vi "Begin.vi"(8 "error in":errorcluster) -> (0 "error out":errorcluster)   [LabVIEW 2015]
doc: "Called before other user functions, this VI is expected to open initial I/O refnums, load in file data, and do all program initialization. Notice that the <B>error out</B> terminal is simply used for data flow. Wiring it to other structures or subVIs ensures that this VI runs first."
uses:
  <vilib>/Rock Robotics/SystemInterfaces/i2clib/i2c_bus.ctl
  <vilib>/Rock Robotics/WPI/I2C/WPI_I2CDevRef.ctl
  <vilib>/Rock Robotics/WPI/DriverStation/WPI_DriverStationRobotMode2.ctl
  <vilib>/Rock Robotics/WPI/Joystick/WPI_JoystickDeviceEnum.ctl
  <vilib>/Rock Robotics/SystemInterfaces/AI/FPGA_AIGyroChannel.ctl
  <vilib>/Rock Robotics/WPI/Accelerometer/WPI_AccelerometerRange.ctl
  <vilib>/Rock Robotics/WPI/Solenoid/WPI_SolenoidChannel.ctl
  <vilib>/Rock Robotics/SystemInterfaces/DIO/FPGA_DIOChannel.ctl
  <vilib>/Rock Robotics/SystemInterfaces/DIO/FPGA_DIOPWMChannel.ctl
  <vilib>/Rock Robotics/SystemInterfaces/AI/FPGA_AIChannel.ctl
  <vilib>/Rock Robotics/WPI/CAN/TalonSRX/WPI_CANTalonSRX_BrakeOverride.ctl
  Robot Global Data.vi
  <vilib>/Rock Robotics/WPI/Gyro/WPI_GyroAnalogOpen.vi
  <vilib>/Rock Robotics/WPI/Accelerometer/InternalAccelerometer/WPI_AccelerometerInternalOpen.vi
  <vilib>/Rock Robotics/WPI/Solenoid/WPI_SolenoidOpenDouble.vi
  <vilib>/Rock Robotics/WPI/Counter/WPI_CounterDigitalInputToDigitalSource.vi
  <vilib>/Rock Robotics/WPI/MotorControl/WPI_MotorControlOpen Talon.vi
  <vilib>/Rock Robotics/WPI/MotorControl/WPI_MotorControlOpenCANTalonSRX.vi
  <vilib>/Rock Robotics/WPI/RobotDrive/WPI_RobotDriveOpen4MotorWithCANTalonSRX.vi
  <vilib>/Rock Robotics/WPI/RobotDrive/WPI_RobotDriveOpen2MotorWithTalon.vi
panel:
  in  "Alt Adr":bool=TRUE
  in  "Flash Drive? 2":bool
  out "I2CDevRef out 2":T1={"DevStatus"={"status"=FALSE, "code"=0, "source"=""}, "Device Address"=40, "Handle"=45, "I2C Bus"=enum."I2C MXP"} {"Device Address" format="%.0x"}
  out "Fatal Result 2":bool
  out "Bad result 2":bool
  in  "Calibrate? 2":bool
  in  "Status delay 2":i32=30
  in  "I2C Bus 2":T2=enum."I2C MXP"
  in  "Placement 2":T3(ring)=enum."P3"
  in  "Op Mode 2":T4(ring)=enum."IMU"
  out "M 2":T5={"Boolean"=TRUE, "Boolean 2"=FALSE, "Boolean 3"=FALSE, "Boolean 4"=FALSE}
  out "A 2":T5={"Boolean"=TRUE, "Boolean 2"=FALSE, "Boolean 3"=FALSE, "Boolean 4"=FALSE}
  out "G 2":T5={"Boolean"=TRUE, "Boolean 2"=FALSE, "Boolean 3"=FALSE, "Boolean 4"=FALSE}
  out "S 2":T5={"Boolean"=TRUE, "Boolean 2"=FALSE, "Boolean 3"=FALSE, "Boolean 4"=FALSE}
  in  "Flash Drive?":bool
  out "I2CDevRef out":T1={"DevStatus"={"status"=FALSE, "code"=0, "source"=""}, "Device Address"=40, "Handle"=45, "I2C Bus"=enum."I2C MXP"} {"Device Address" format="%.0x"}
  out "Fatal Result":bool
  out "Bad result":bool
  out "M":T5={"Boolean"=TRUE, "Boolean 2"=FALSE, "Boolean 3"=FALSE, "Boolean 4"=FALSE}
  out "A":T5={"Boolean"=TRUE, "Boolean 2"=FALSE, "Boolean 3"=FALSE, "Boolean 4"=FALSE}
  out "G":T5={"Boolean"=TRUE, "Boolean 2"=FALSE, "Boolean 3"=FALSE, "Boolean 4"=FALSE}
  out "S":T5={"Boolean"=TRUE, "Boolean 2"=FALSE, "Boolean 3"=FALSE, "Boolean 4"=FALSE}
  in  "Calibrate?":bool
  in  "Status delay":i32=30
  in  "I2C Bus":T2=enum."I2C MXP"
  in  "Placement":T3(ring)=enum."P3"
  in  "Op Mode":T4(ring)=enum."IMU"
  # "C-BOT:"
  # "BNO055 Cal MC P3 01-29-2016 142659"
  # "Alt IMU CBOT CHAMPS: BNO055 Cal M8 P3 04-27-2016 180927"
  # "P-BOT;"
  # "BNO055 Cal MC P3 02-26-2016 205524"
  # "CBOT CHAMPS Pri: BNO055 Cal M8 P3 04-27-2016 181522"
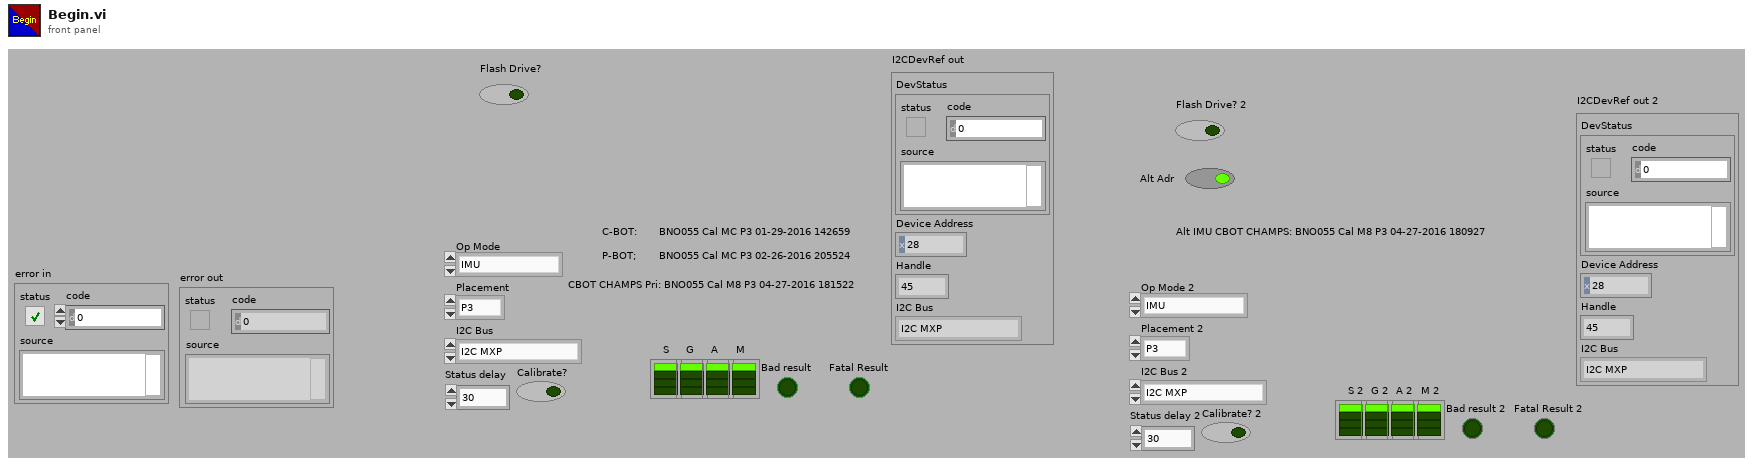
[diagram p1: front panel]
types:
  T1 = typedef "WPI_I2CDevRef.ctl" = cluster{"DevStatus":errorcluster, "Device Address":u8, "Handle":i32, "I2C Bus":T2}
  T2 = typedef "i2c_bus.ctl" = enum16{"I2C On-Board", "I2C MXP", "Invalid"}
  T3 = enum32{"P0", "P1", "P2", "P3", "P4", "P5", "P6", "P7"}
  T4 = enum8{"ConfigMode", "AccOnly", "MagOnly", "GyroOnly", "AccMag", "AccGyro", "MagGyro", "AMG", "IMU", "Compass", "M4G", "NDOF_FMC_OFF", "NDOF"}
  T5 = cluster{"Boolean":bool, "Boolean 2":bool, "Boolean 3":bool, "Boolean 4":bool}
  T6 = typedef "FPGA_DIOPWMChannel.ctl" = enum8{"PWM 0", "PWM 1", "PWM 2", "PWM 3", "PWM 4", "PWM 5", "PWM 6", "PWM 7", "PWM 8", "PWM 9", "PWM MXP 0", "PWM MXP 1", "PWM MXP 2", "PWM MXP 3", "PWM MXP 4", "PWM MXP 5", "PWM MXP 6", "PWM MXP 7", "PWM MXP 8", "PWM MXP 9", "Invalid"}
  T7 = typedef "WPI_SolenoidChannel.ctl" = enum8{"Solenoid 0", "Solenoid 1", "Solenoid 2", "Solenoid 3", "Solenoid 4", "Solenoid 5", "Solenoid 6", "Solenoid 7", "Invalid"}
  T8 = typedef "FPGA_AIChannel.ctl" = enum8{"AI 0", "AI 1", "AI 2", "AI 3", "AI MXP 0", "AI MXP 1", "AI MXP 2", "AI MXP 3", "Invalid"}
  T9 = typedef "FPGA_AIGyroChannel.ctl" = enum8{"AI 0", "AI 1", "Invalid"}
  T10 = typedef "WPI_JoystickDeviceEnum.ctl" = enum16{"USB 0", "USB 1", "USB 2", "USB 3", "USB 4", "USB 5"}
  T11 = typedef "FPGA_DIOChannel.ctl" = enum8{"DIO 0", "DIO 1", "DIO 2", "DIO 3", "DIO 4", "DIO 5", "DIO 6", "DIO 7", "DIO 8", "DIO 9", "DIO MXP 0", "DIO MXP 1", "DIO MXP 2", "DIO MXP 3", "DIO MXP 4", "DIO MXP 5", "DIO MXP 6", "DIO MXP 7", "DIO MXP 8", "DIO MXP 9", "DIO MXP 10", "DIO MXP 11", "DIO MXP 12", "DIO MXP 13", "DIO MXP 14", "DIO MXP 15", "Invalid"}
  T12 = typedef "WPI_AccelerometerRange.ctl" = enum16{"+/- 2 g", "+/- 4 g", "+/- 8 g"}
  T13 = typedef "WPI_DriverStationRobotMode2.ctl" = enum16{"Autonomous Disabled", "Autonomous Enabled", "Teleop Disabled", "Teleop Enabled", "Disconnected", "Finish", "Test Disabled", "Test Enabled", "Emergency Stopped"}
  T14 = typedef "WPI_CANTalonSRX_BrakeOverride.ctl" = enum8{"No Override", "Override to Coast", "Override to Brake"}
  T15 = typedef "WPI_MotorControlDeviceRef.ctl" = cluster{"DeviceStatus":errorcluster, "Type":T16, "PWM":cluster{"PWM Channel":T6, "DeadBand":T17}, "CAN":cluster{"Device Number":u8, "Control Mode":T18, "Semaphore":T19, "Max Vout":dbl, "TalonSRX Control Mode":T20}, "Invert":bool}
  T16 = typedef "WPI_MotorControlType.ctl" = enum16{"PWM", "CAN", "CANTalonSRX"}
  T17 = typedef "WPI_PWMDeadband.ctl" = cluster{"Name":string, "maxPositivePwm":i32, "minPositivePwm":i32, "centerPwm":i32, "maxNegativePwm":i32, "minNegativePwm":i32, "angularRange":u16}
  T18 = typedef "WPI_CANJaguar_ControlMode.ctl" = enum8{"Percent VBus", "Current", "Speed", "Position", "Voltage"}
  T19 = typedef "Semaphore RefNum" = refnum<k1>
  T20 = typedef "WPI_CANTalonSRX_APIControlMode.ctl" = enum8{"Percent VBus", "Speed", "Position", "Slave", "Unchanged / Invalid", "Voltage Compensation", "Current", "Motion Profile"}
  T21 = typedef "WPI_RobotDriveDevRef.ctl" = cluster{"DevStatus":errorcluster, "Motors[]":T15[], "Square Inputs":bool, "Max Output":dbl}
  T22 = typedef "WPI_AccelerometerDevRef.ctl" = cluster{"DevStatus":errorcluster, "Scaling":T23, "Analog Channels":T24, "I2C Bus":T2, "SPI Bus":T25, "Accel Range":T26, "ADXL Axes":T27, "Handle":i32, "Device Address":u8, "Accel Type":enum16{"Analog", "ADXL345 I2C", "ADXL345 SPI", "Internal", "ADXL362 SPI"}}
  T23 = typedef "WPI_AccelerometerScaling.ctl" = cluster{"Gain (VoltsPerG)":dbl, "Center Voltage":dbl}
  T24 = typedef "WPI_AccelerometerAnalogChannels.ctl" = cluster{"X-Axis":T8, "Y-Axis":T8, "Z-Axis":T8}
  T25 = typedef "spi_bus.ctl" = enum16{"SPI On-Board, CS0", "SPI On-Board, CS1", "SPI On-Board, CS2", "SPI On-Board, CS3", "SPI MXP", "Invalid"}
  T26 = typedef "ADXL345 Range.ctl" = u8
  T27 = typedef "WPI_AccelerometerADXL345 Axes.ctl" = cluster{"X-Axis":bool, "Y-Axis":bool, "Z-Axis":bool}
  T28 = typedef "WPI_DigitalInputDevRef.ctl" = cluster{"DevStatus":errorcluster, "DIO Channel":T11}
  T29 = typedef "FPGA_CounterEncoderSourceConvertionLVSourceType.ctl" = cluster{"DevStatus":errorcluster, "AnalogTriggerMode?":bool, "DigitalMode":cluster{"DIO Channel":T30}, "AnalogTriggerMode":cluster{"AnalogTriggerIndex":T31, "OutputType":T32}}
  T30 = typedef "FPGA_DIODigitalSourceChannel.ctl" = enum8{"DIO 0", "DIO 1", "DIO 2", "DIO 3", "DIO 4", "DIO 5", "DIO 6", "DIO 7", "DIO 8", "DIO 9", "DIO MXP 0", "DIO MXP 1", "DIO MXP 2", "DIO MXP 3", "DIO MXP 4", "DIO MXP 5", "DIO MXP 6", "DIO MXP 7", "DIO MXP 8", "DIO MXP 9", "DIO MXP 10", "DIO MXP 11", "DIO MXP 12", "DIO MXP 13", "DIO MXP 14", "DIO MXP 15", "Disabled"}
  T31 = typedef "FPGA_AnalogTriggerIndex.ctl" = enum8{"Trig 0", "Trig 1", "Trig 2", "Trig 3", "Trig 4", "Trig 5", "Trig 6", "Trig 7", "Invalid"}
  T32 = typedef "FPGA_AnalogTriggerOutType.ctl" = enum16{"InWindow", "TriggerState", "Rising", "Falling"}
  T33 = typedef "WPI_EncoderDevRef.ctl" = cluster{"DevStatus":errorcluster, "EncoderIndex":T34, "CounterIndex":T35, "DistancePerCount":dbl, "Decoding Type":T36}
  T34 = typedef "FPGA_EncoderIdx.ctl" = enum8{"Enc 0", "Enc 1", "Enc 2", "Enc 3", "Enc 4", "Enc 5", "Enc 6", "Enc 7", "Invalid"}
  T35 = typedef "FPGA_CounterCtrSystemIndex.ctl" = enum8{"Ctr 0", "Ctr 1", "Ctr 2", "Ctr 3", "Ctr 4", "Ctr 5", "Ctr 6", "Ctr 7", "Invalid"}
  T36 = typedef "WPI_EncoderType.ctl" = enum16{"1x", "2x", "4x"}
  T37 = cluster{"Cluster":cluster{"[0]":bool, "[1]":bool, "[2]":bool, "[3]":bool}, "Cluster":cluster{"[0]":bool, "[1]":bool, "[2]":bool, "[3]":bool}, "Cluster":cluster{"[0]":bool, "[1]":bool, "[2]":bool, "[3]":bool}, "Cluster":cluster{"[0]":bool, "[1]":bool, "[2]":bool, "[3]":bool}}
  T38 = cluster{"[0]":bool, "[1]":bool, "[2]":bool, "[3]":bool}
  T39 = typedef "WPI_JoystickDevRef.ctl" = cluster{"Device":T10}
  T40 = typedef "WPI_SolenoidDevRef.ctl" = cluster{"DevStatus":errorcluster, "Pneumatics Control Module":u8, "Forward Solenoid Channel":T7, "Reverse Solenoid Channel":T7}
  T41 = typedef "WPI_GyroDevRef.ctl" = cluster{"DevStatus":errorcluster, "Analog Channel":T8, "Offset":dbl, "Gain (VoltsPerDegree/Second)":dbl, "Gyro Type":enum16{"Analog", "XRS450"}, "Handle":i32, "SPI Bus":T25, "Device Found":bool, "Sample Rate":dbl, "Calibrate On Open":bool}
  T42 = typedef "WPI_ServoDeviceRef.ctl" = cluster{"DeviceStatus":errorcluster, "PWM Channel":T6, "DeadBand":T17}
  T43 = typedef "WPI_AnalogChannelDevRef.ctl" = cluster{"DevStatus":errorcluster, "Analog Channel":T8}
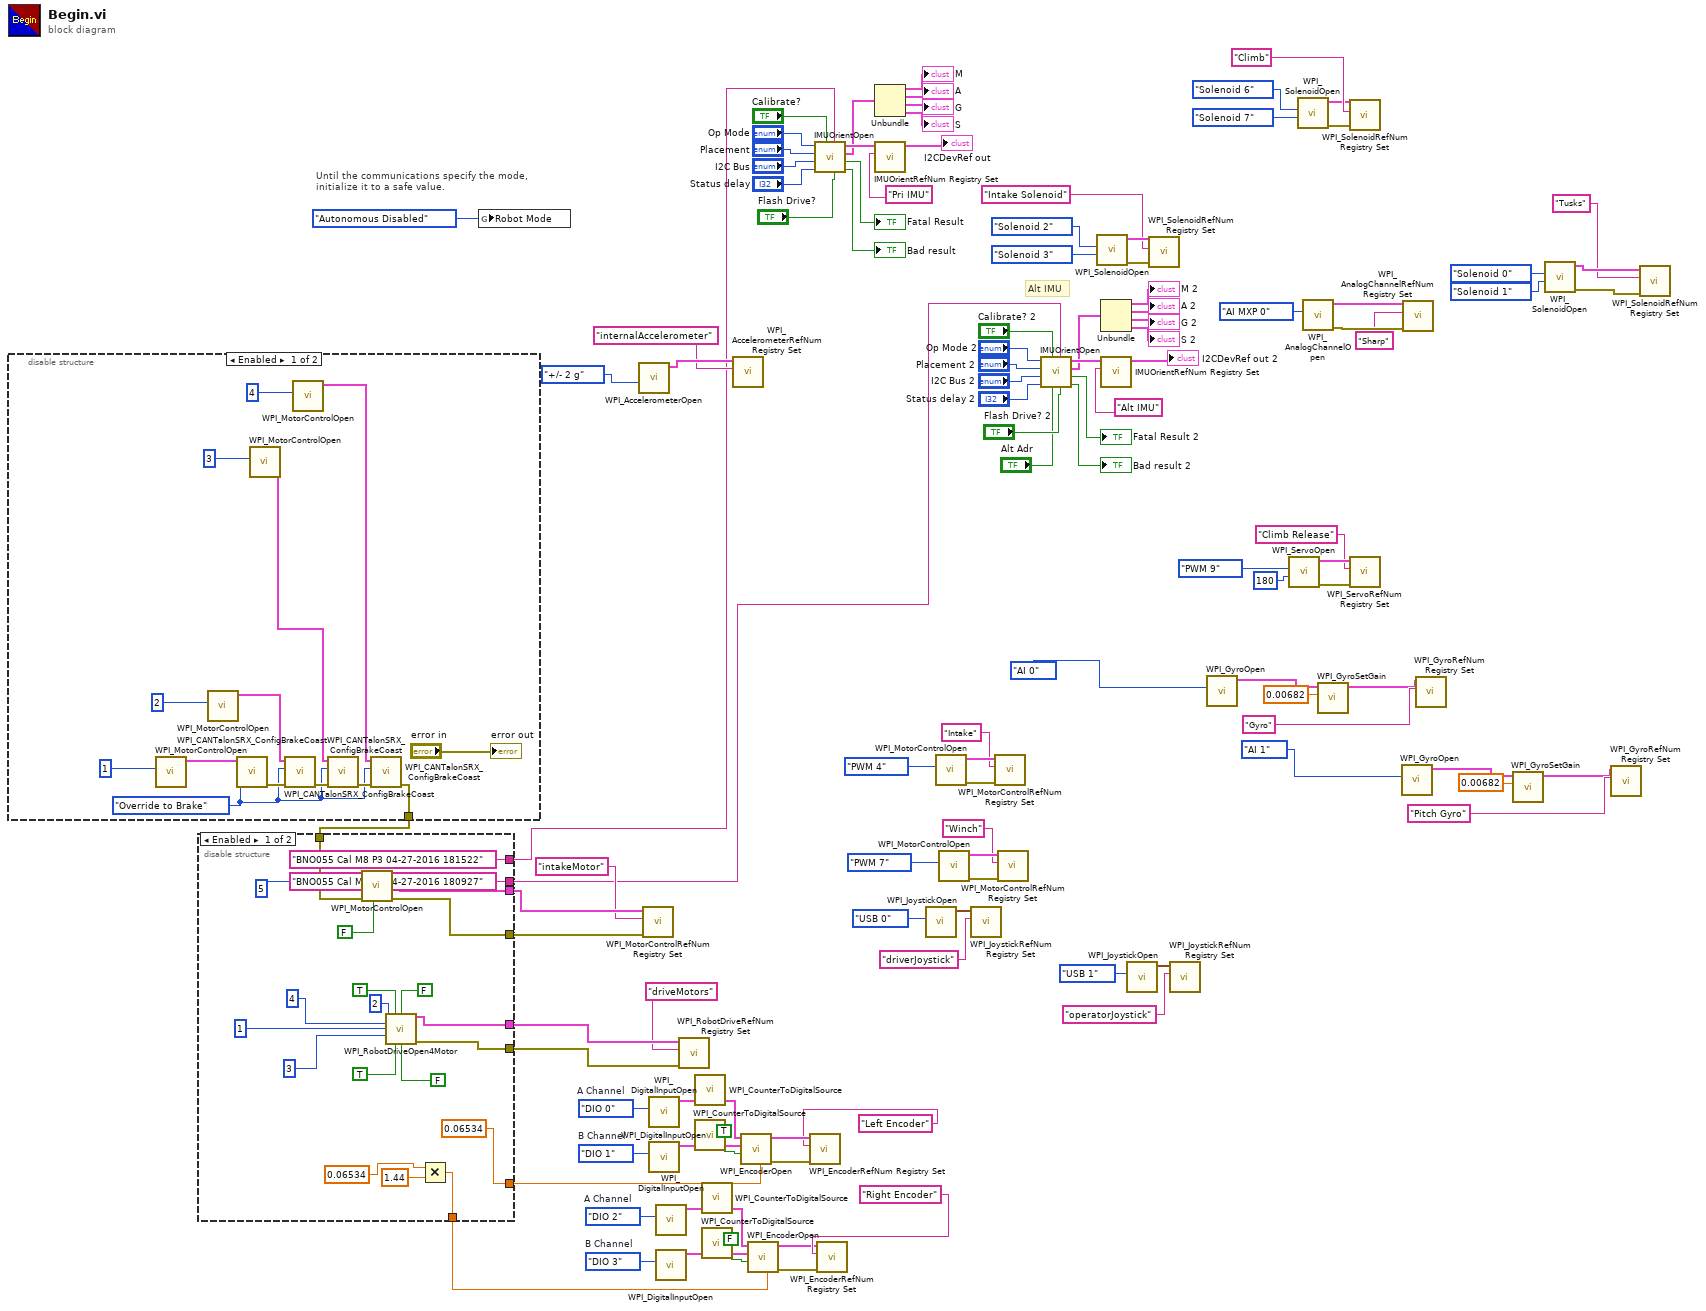
[diagram p0: block diagram]
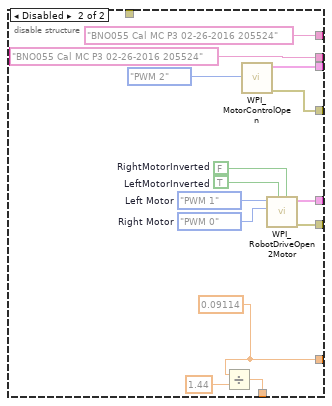
[diagram p3: hidden frame]
diagram:
  w62 = FPGA_DIOChannel."DIO 3"  # B Channel
  w63 = FPGA_DIOChannel."DIO 2"  # A Channel
  w79 = FPGA_DIOChannel."DIO 1"  # B Channel
  w78 = FPGA_DIOChannel."DIO 0"  # A Channel
  # "Alt IMU"
  # "Until the communications specify the mode,\ninitialize it to a safe value."
  n1 = disable-structure shown="Enabled" {
    disable-tunnel: [w129 _] -> w53
    frame Enabled {
      w117 = WPI_CANTalonSRX_BrakeOverride."Override to Brake" ("Brake / Coast Mode")
      n2 = call-poly <vilib>:"WPI_MotorControlOpen.vi"("Device Number"=u8 1) -> ("MotorControlDeviceRef"=w122:T15)  [unwired: 9 in, 1 out]
      n3 = call-poly <vilib>:"WPI_MotorControlOpen.vi"("Device Number"=u8 2) -> ("MotorControlDeviceRef"=w123:T15)  [unwired: 9 in, 1 out]
      n4 = call <vilib>:"WPI_CANTalonSRX_ConfigBrakeCoast.vi"("Brake / Coast Mode"=w117, "CAN Talon SRX Ref"=w122) -> ("error out"=w128:errorcluster)  [unwired: 8 in, 1 out]
      n5 = call-poly <vilib>:"WPI_MotorControlOpen.vi"("Device Number"=u8 3) -> ("MotorControlDeviceRef"=w124:T15)  [unwired: 9 in, 1 out]
      n6 = call <vilib>:"WPI_CANTalonSRX_ConfigBrakeCoast.vi"("error in (no error)"=w128, "Brake / Coast Mode"=w117, "CAN Talon SRX Ref"=w123) -> ("error out"=w127:errorcluster)  [unwired: 7 in, 1 out]
      n7 = call-poly <vilib>:"WPI_MotorControlOpen.vi"("Device Number"=u8 4) -> ("MotorControlDeviceRef"=w125:T15)  [unwired: 9 in, 1 out]
      n8 = call <vilib>:"WPI_CANTalonSRX_ConfigBrakeCoast.vi"("error in (no error)"=w127, "Brake / Coast Mode"=w117, "CAN Talon SRX Ref"=w124) -> ("error out"=w126:errorcluster)  [unwired: 7 in, 1 out]
      n9 = call <vilib>:"WPI_CANTalonSRX_ConfigBrakeCoast.vi"("error in (no error)"=w126, "Brake / Coast Mode"=w117, "CAN Talon SRX Ref"=w125) -> ("error out"=w129:errorcluster)  [unwired: 7 in, 1 out]
      "error out" <- "error in"
    }
    frame Disabled {
    }
  }
  n10 = disable-structure shown="Enabled" {
    disable-tunnel: [w147 w163] -> w116
    disable-tunnel: [w148 w162] -> w114
    disable-tunnel: [w151 w158] -> w86
    disable-tunnel: [w150 w157] -> w54
    disable-tunnel: w53 -> [w137 _]
    disable-tunnel: [w134 w154] -> w52
    disable-tunnel: [0.06534 ("DistancePerCount") w156] -> w51
    disable-tunnel: ["BNO055 Cal M8 P3 04-27-2016 181522" ("Stored Cal File") "BNO055 Cal MC P3 02-26-2016 205524" ("Stored Cal File")] -> w30
    disable-tunnel: ["BNO055 Cal M8 P3 04-27-2016 180927" ("Stored Cal File") "BNO055 Cal MC P3 02-26-2016 205524" ("Stored Cal File")] -> w1
    frame Enabled {
      n11 = call-poly <vilib>:"WPI_MotorControlOpen.vi"("Invert"=FALSE, "error in (no error)"=w137, "Device Number"=u8 5) -> ("error out"=w150:errorcluster, "MotorControlDeviceRef"=w151:T15)  [unwired: 7 in]
      n12 = call-poly <vilib>:"WPI_RobotDriveOpen4Motor.vi"("Rear Left Motor"=u8 2, "Rear Left Motor Inverted"=TRUE, "Rear Right Motor Inverted"=FALSE, "Rear Right Motor"=u8 4, "Front Left Motor"=u8 1, "Front Right Motor"=u8 3, "Front Left Motor Inverted"=TRUE, "Front Right Motor Inverted"=FALSE) -> ("RobotDriveDevRef"=w147:T21, "error out"=w148:errorcluster)  [unwired: 6 in]
      n13 = Multiply(x=0.06534 ("DistancePerCount"), y=1.44) -> (x*y=w134:dbl)
    }
    frame Disabled {
      w156 = 0.09114 ("DistancePerCount")
      w160 = FPGA_DIOPWMChannel."PWM 0"  # Right Motor
      w161 = FPGA_DIOPWMChannel."PWM 1"  # Left Motor
      w164 = TRUE  # LeftMotorInverted
      w165 = FALSE  # RightMotorInverted
      n14 = Divide(x=w156, y=1.44) -> (x/y=w154:dbl)
      n15 = call-poly <vilib>:"WPI_MotorControlOpen.vi"("PWM Channel"=FPGA_DIOPWMChannel."PWM 2") -> ("error out"=w157:errorcluster, "MotorControlDeviceRef"=w158:T15)  [unwired: 9 in]
      n16 = call-poly <vilib>:"WPI_RobotDriveOpen2Motor.vi"("Right Motor Inverted"=w165, "Left Motor Inverted"=w164, "Right Motor"=w160, "Left Motor"=w161) -> ("error out"=w162:errorcluster, "RobotDriveDevRef"=w163:T21)  [unwired: 1 in, 5 out]
    }
  }
  n17 = global write "Robot Global Data.vi" "Robot Mode"(WPI_DriverStationRobotMode2."Autonomous Disabled" ("Robot Mode")) -> ()
  n18 = call-poly <vilib>:"WPI_AccelerometerOpen.vi"("Accel Range"=WPI_AccelerometerRange."+/- 2 g") -> ("AccelerometerDevRef"=w90:T22)  [unwired: 9 in, 1 out]
  n19 = call <vilib>:"WPI_MotorControlRefNum Registry Set.vi"("error in (no error)"=w54, "refnum name"="intakeMotor", "MotorControlDevRef"=w86) -> ()  [unwired: 7 in, 2 out]
  n20 = call <vilib>:"WPI_DigitalInputOpen.vi"("DIO Channel"=w78) -> ("DigitalInputDevRef"=w75:T28)  [unwired: 1 in, 9 out]
  n21 = call <vilib>:"WPI_DigitalInputOpen.vi"("DIO Channel"=w79) -> ("DigitalInputDevRef"=w76:T28)  [unwired: 1 in, 9 out]
  n22 = call <vilib>:"WPI_DigitalInputOpen.vi"("DIO Channel"=w63) -> ("DigitalInputDevRef"=w66:T28)  [unwired: 1 in, 9 out]
  n23 = call <vilib>:"WPI_DigitalInputOpen.vi"("DIO Channel"=w62) -> ("DigitalInputDevRef"=w65:T28)  [unwired: 1 in, 9 out]
  n24 = call <vilib>:"WPI_RobotDriveRefNum Registry Set.vi"("error in (no error)"=w114, "refnum name"="driveMotors", "RobotDriveDevRef"=w116) -> ()  [unwired: 1 in, 8 out]
  n25 = call-poly <vilib>:"WPI_CounterToDigitalSource.vi"("DigitalInputDevRef"=w75) -> ("Digital Source"=w74:T29)  [unwired: 6 out]
  n26 = call-poly <vilib>:"WPI_CounterToDigitalSource.vi"("DigitalInputDevRef"=w76) -> ("Digital Source"=w77:T29)  [unwired: 6 out]
  n27 = call-poly <vilib>:"WPI_CounterToDigitalSource.vi"("DigitalInputDevRef"=w66) -> ("Digital Source"=w67:T29)  [unwired: 6 out]
  n28 = call-poly <vilib>:"WPI_CounterToDigitalSource.vi"("DigitalInputDevRef"=w65) -> ("Digital Source"=w64:T29)  [unwired: 6 out]
  n29 = call <vilib>:"WPI_AccelerometerRefNum Registry Set.vi"("refnum name"="internalAccelerometer", "AccelerometerDevRef"=w90) -> ()  [unwired: 8 in, 2 out]
  n30 = call <vilib>:"WPI_EncoderOpen.vi"("DistancePerCount"=w51, "Invert Direction (False)"=TRUE, "BSource"=w77, "ASource"=w74) -> ("error out"=w72:errorcluster, "EncoderDevRef"=w73:T33)  [unwired: 4 in, 2 out]
  n31 = call <vilib>:"WPI_EncoderOpen.vi"("DistancePerCount"=w52, "Invert Direction (False)"=FALSE, "BSource"=w64, "ASource"=w67) -> ("error out"=w69:errorcluster, "EncoderDevRef"=w68:T33)  [unwired: 4 in, 2 out]
  n32 = call <vilib>:"WPI_EncoderRefNum Registry Set.vi"("error in (no error)"=w72, "refnum name"="Left Encoder", "EncoderDevRef"=w73) -> ()  [unwired: 7 in, 2 out]
  n33 = call "IMUOrientOpen.vi"("Flash Drive?"="Flash Drive?", "Stored Cal File"=w30, "Calibrate?"="Calibrate?", "Status delay"="Status delay", "I2C Bus"="I2C Bus", "Placement"="Placement", "Op Mode"="Op Mode") -> ("Bad result"=→"Bad result":bool, "Fatal Result"=→"Fatal Result":bool, "Cal Status"=w93:T37, "I2CDevRef"=w100:T1)  [unwired: 1 in]
  n34 = call <vilib>:"WPI_EncoderRefNum Registry Set.vi"("error in (no error)"=w69, "refnum name"="Right Encoder", "EncoderDevRef"=w68) -> ()  [unwired: 7 in, 2 out]
  n35 = Unbundle(w93) -> ("Cluster"=→"M":T38, "Cluster"=→"A":T38, "Cluster"=→"G":T38, "Cluster"=→"S":T38)
  n36 = call "IMUOrientRefNum Registry Set.vi"("refnum name"="Pri IMU", "I2CDevRef in"=w100) -> ("I2CDevRef out"=→"I2CDevRef out":T1)  [unwired: 8 in, 1 out]
  n37 = call <vilib>:"WPI_JoystickOpen.vi"("JoystickDevice"=WPI_JoystickDeviceEnum."USB 0") -> ("JoystickDevRef"=w111:T39)  [unwired: 10 in]
  n38 = call-poly <vilib>:"WPI_MotorControlOpen.vi"("PWM Channel"=FPGA_DIOPWMChannel."PWM 4") -> ("error out"=w46:errorcluster, "MotorControlDeviceRef"=w47:T15)  [unwired: 9 in]
  n39 = call-poly <vilib>:"WPI_MotorControlOpen.vi"("PWM Channel"=FPGA_DIOPWMChannel."PWM 7") -> ("error out"=w42:errorcluster, "MotorControlDeviceRef"=w41:T15)  [unwired: 9 in]
  n40 = call <vilib>:"WPI_JoystickRefNum Registry Set.vi"("refnum name"="driverJoystick", "JoystickDevRef"=w111) -> ()  [unwired: 8 in, 2 out]
  n41 = call <vilib>:"WPI_MotorControlRefNum Registry Set.vi"("error in (no error)"=w46, "refnum name"="Intake", "MotorControlDevRef"=w47) -> ()  [unwired: 7 in, 2 out]
  n42 = call <vilib>:"WPI_MotorControlRefNum Registry Set.vi"("error in (no error)"=w42, "refnum name"="Winch", "MotorControlDevRef"=w41) -> ()  [unwired: 7 in, 2 out]
  n43 = call "IMUOrientOpen.vi"("Flash Drive?"="Flash Drive? 2", "Stored Cal File"=w1, "Alt Adr"="Alt Adr", "Calibrate?"="Calibrate? 2", "Status delay"="Status delay 2", "I2C Bus"="I2C Bus 2", "Placement"="Placement 2", "Op Mode"="Op Mode 2") -> ("Bad result"=→"Bad result 2":bool, "Fatal Result"=→"Fatal Result 2":bool, "Cal Status"=w7:T37, "I2CDevRef"=w14:T1)
  n44 = call-poly <vilib>:"WPI_SolenoidOpen.vi"("Reverse Solenoid Channel"=WPI_SolenoidChannel."Solenoid 3", "Forward Solenoid Channel"=WPI_SolenoidChannel."Solenoid 2") -> ("error out"=w82:errorcluster, "SolenoidDevRef"=w81:T40)  [unwired: 8 in]
  n45 = Unbundle(w7) -> ("Cluster"=→"M 2":T38, "Cluster"=→"A 2":T38, "Cluster"=→"G 2":T38, "Cluster"=→"S 2":T38)
  n46 = call "IMUOrientRefNum Registry Set.vi"("refnum name"="Alt IMU", "I2CDevRef in"=w14) -> ("I2CDevRef out"=→"I2CDevRef out 2":T1)  [unwired: 8 in, 1 out]
  n47 = call <vilib>:"WPI_JoystickOpen.vi"("JoystickDevice"=WPI_JoystickDeviceEnum."USB 1") -> ("JoystickDevRef"=w49:T39)  [unwired: 10 in]
  n48 = call <vilib>:"WPI_SolenoidRefNum Registry Set.vi"("error in (no error)"=w82, "refnum name"="Intake Solenoid", "SolenoidDevRef"=w81) -> ()  [unwired: 7 in, 2 out]
  n49 = call <vilib>:"WPI_JoystickRefNum Registry Set.vi"("refnum name"="operatorJoystick", "JoystickDevRef"=w49) -> ()  [unwired: 8 in, 2 out]
  n50 = call-poly <vilib>:"WPI_GyroOpen.vi"("Analog Channel"=FPGA_AIGyroChannel."AI 0") -> ("GyroDevRef"=w107:T41)  [unwired: 8 in, 2 out]
  n51 = call <vilib>:"WPI_ServoOpen.vi"("Angular Range"=u16 180, "PWM Channel"=FPGA_DIOPWMChannel."PWM 9") -> ("error out"=w22:errorcluster, "ServoDeviceRef"=w21:T42)  [unwired: 8 in]
  n52 = call-poly <vilib>:"WPI_SolenoidOpen.vi"("Reverse Solenoid Channel"=WPI_SolenoidChannel."Solenoid 7", "Forward Solenoid Channel"=WPI_SolenoidChannel."Solenoid 6") -> ("error out"=w27:errorcluster, "SolenoidDevRef"=w28:T40)  [unwired: 8 in]
  n53 = call <vilib>:"WPI_AnalogChannelOpen.vi"("Analog Channel"=FPGA_AIChannel."AI MXP 0") -> ("error out"=w33:errorcluster, "AIDeviceRef"=w34:T43)  [unwired: 9 in]
  n54 = call <vilib>:"WPI_GyroSetGain.vi"("Gain (VoltsPerDegree/Second)"=0.00682, "GyroDevRef"=w107) -> ("GyroDevRef"=w106:T41)  [unwired: 8 in, 1 out]
  n55 = call <vilib>:"WPI_SolenoidRefNum Registry Set.vi"("error in (no error)"=w27, "refnum name"="Climb", "SolenoidDevRef"=w28) -> ()  [unwired: 7 in, 2 out]
  n56 = call <vilib>:"WPI_ServoRefNum Registry Set.vi"("error in (no error)"=w22, "refnum name"="Climb Release", "ServoDeviceRef"=w21) -> ()  [unwired: 7 in, 2 out]
  n57 = call-poly <vilib>:"WPI_GyroOpen.vi"("Analog Channel"=FPGA_AIGyroChannel."AI 1") -> ("GyroDevRef"=w38:T41)  [unwired: 8 in, 2 out]
  n58 = call <vilib>:"WPI_AnalogChannelRefNum Registry Set.vi"("error in (no error)"=w33, "refnum name"="Sharp", "AIDeviceRef"=w34) -> ()  [unwired: 7 in, 2 out]
  n59 = call <vilib>:"WPI_GyroRefNum Registry Set.vi"("refnum name"="Gyro", "GyroDevRef"=w106) -> ()  [unwired: 8 in, 2 out]
  n60 = call <vilib>:"WPI_GyroSetGain.vi"("Gain (VoltsPerDegree/Second)"=0.00682, "GyroDevRef"=w38) -> ("GyroDevRef"=w37:T41)  [unwired: 8 in, 1 out]
  n61 = call-poly <vilib>:"WPI_SolenoidOpen.vi"("Reverse Solenoid Channel"=WPI_SolenoidChannel."Solenoid 1", "Forward Solenoid Channel"=WPI_SolenoidChannel."Solenoid 0") -> ("error out"=w58:errorcluster, "SolenoidDevRef"=w59:T40)  [unwired: 8 in]
  n62 = call <vilib>:"WPI_GyroRefNum Registry Set.vi"("refnum name"="Pitch Gyro", "GyroDevRef"=w37) -> ()  [unwired: 8 in, 2 out]
  n63 = call <vilib>:"WPI_SolenoidRefNum Registry Set.vi"("error in (no error)"=w58, "refnum name"="Tusks", "SolenoidDevRef"=w59) -> ()  [unwired: 7 in, 2 out]
